vi "syncAIandAOat1MHz.vi"() -> ()   [LabVIEW 2015]
uses:
  <vilib>/DAQmx/write.llb/DAQmx Write (Digital 1D Wfm NChan NSamp).vi
  <vilib>/DAQmx/write.llb/DAQmx Write (Analog 1D Wfm NChan NSamp).vi
  <vilib>/DAQmx/read.llb/DAQmx Read (Analog 2D I16 NChan NSamp).vi
  <vilib>/Waveform/DWDTOps.llb/DWDT Analog to Digital.vi
  <vilib>/DAQmx/create/channels.llb/DAQmx Create Channel (AO-Voltage-Basic).vi
  <vilib>/DAQmx/create/channels.llb/DAQmx Create Channel (AI-Voltage-Basic).vi
  <vilib>/DAQmx/create/channels.llb/DAQmx Create Channel (DO-Digital Output).vi
  <vilib>/DAQmx/configure/timing.llb/DAQmx Timing (Sample Clock).vi
  <vilib>/Waveform/DWDTOps.llb/DWDT Uncompress Digital.vi
  <vilib>/DAQmx/miscellaneous.llb/DAQmx Fill In Error Info.vi
  <vilib>/DAQmx/configure/trigger.llb/DAQmx Start Trigger (Digital Edge).vi
  <resource>/objmgr/daqmx.rc
panel:
  in  "error in 3":errorcluster caption="error in"
  in  "index (page)":i32
  out "XY Graph":T1(graph)
  in  "V":dbl=2.0 format="%#_13g"
  in  "AOrate":dbl=400000.0 format="%#_13g"
  in  "stop":bool
  out "Intensity Graph":sgl[][](graph)
  in  "error in 2":errorcluster caption="error in"
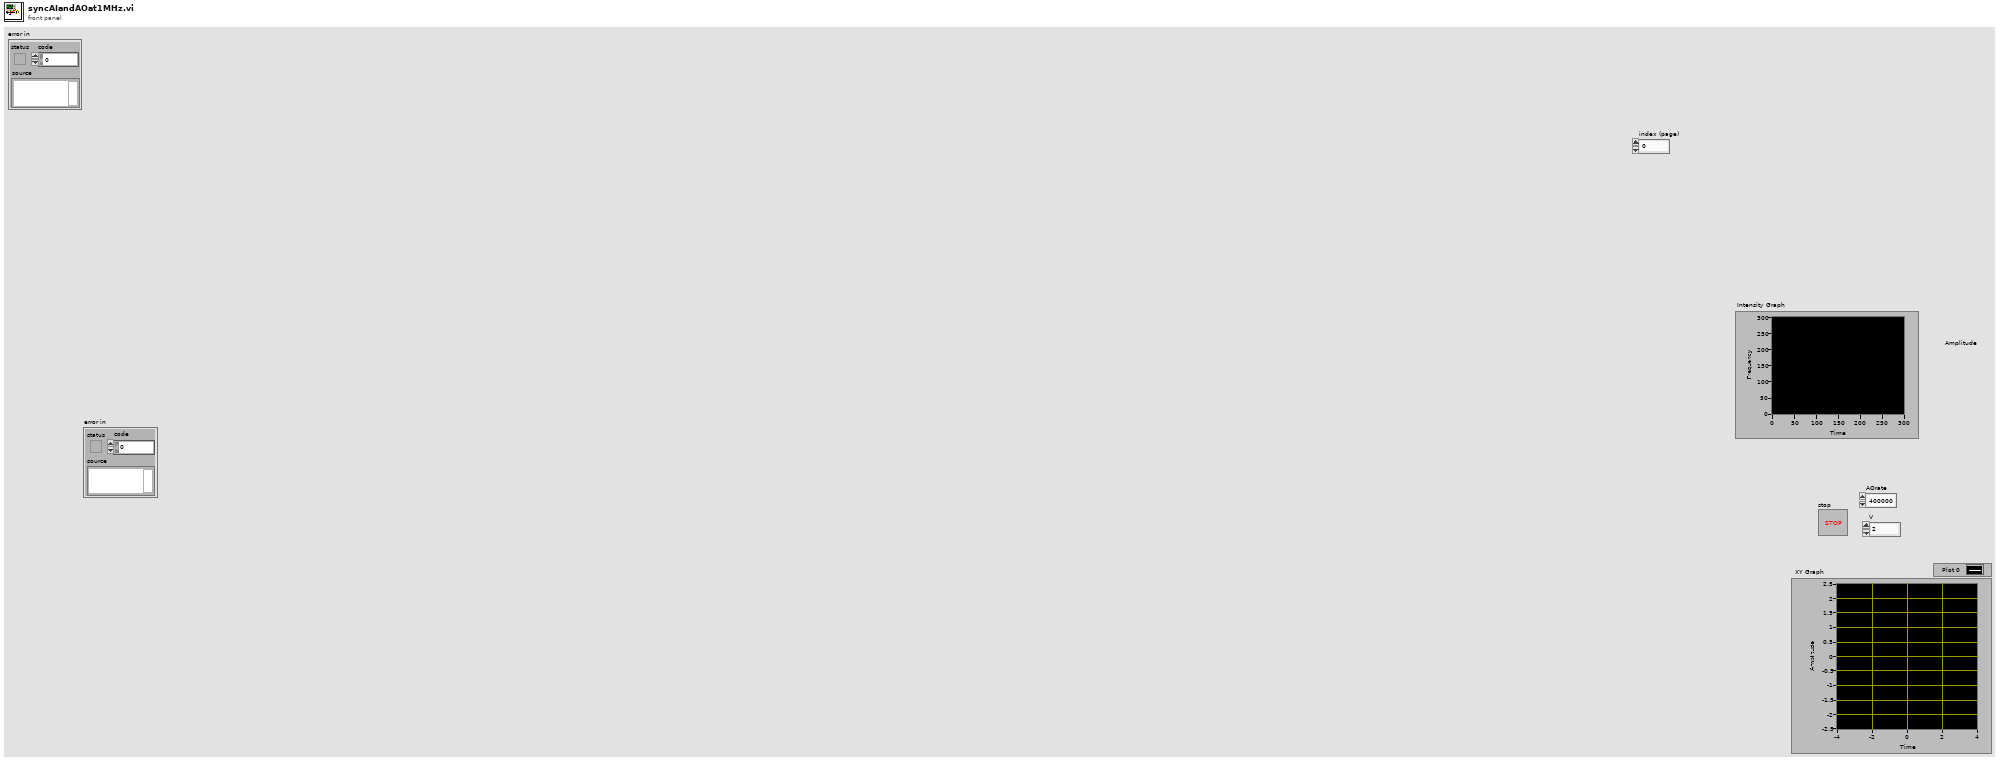
[diagram p1: front panel]
types:
  T1 = cluster{"X-WaveArray":dbl[], "Y-WaveArray":dbl[]}
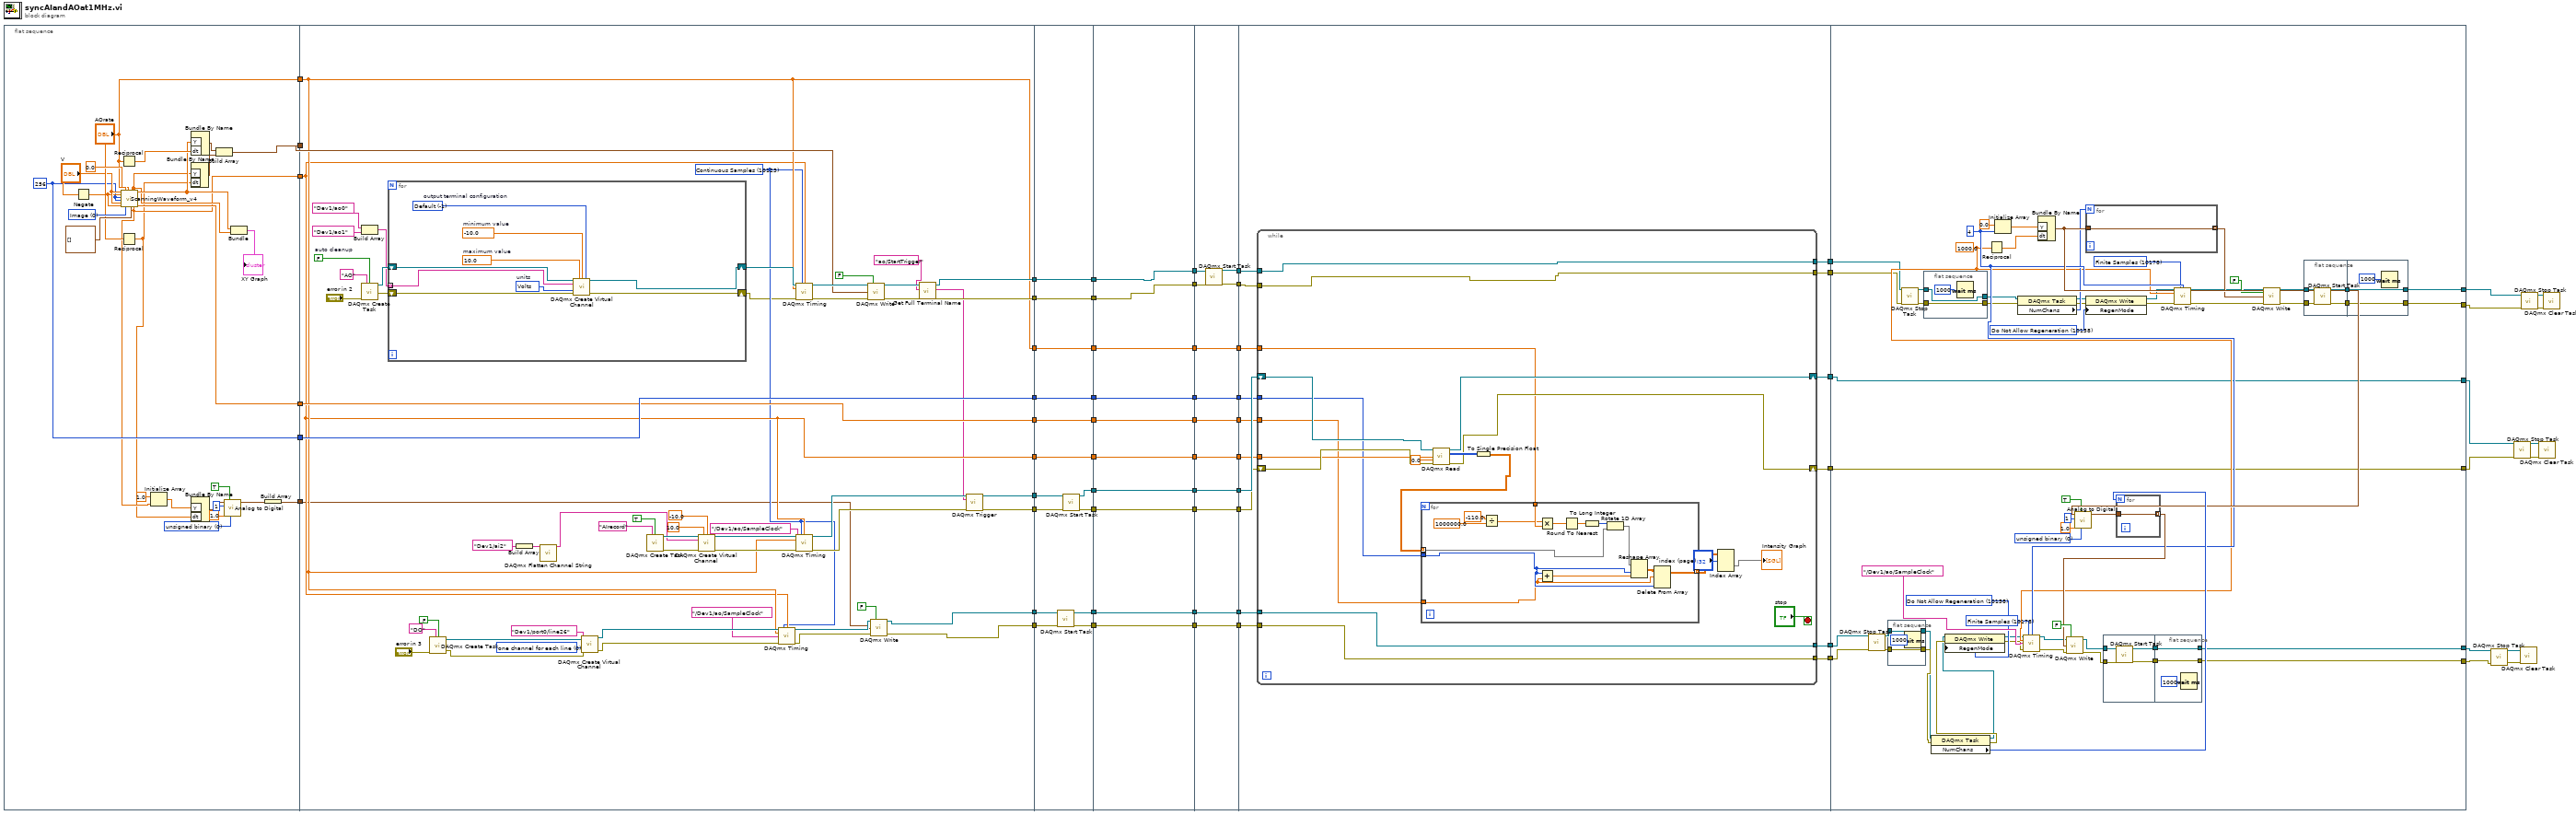
[diagram p0: block diagram]
diagram:
  n1 = flat-sequence {
    tunnel: [w79] -> w64
    tunnel: [w75] -> w63
    tunnel: ["AOrate"] -> w62
    tunnel: [w81] -> w38
    tunnel: [w80] -> w33
    tunnel: [w65] -> w17
    tunnel: w64 -> [w135]
    tunnel: w63 -> [w102]
    tunnel: w62 -> [w103]
    tunnel: [w117] -> w61
    tunnel: [w123] -> w58
    tunnel: [w121] -> w57
    tunnel: [w102] -> w43
    tunnel: [w103] -> w39
    tunnel: w38 -> [w125]
    tunnel: [w125] -> w34
    tunnel: w33 -> [w124]
    tunnel: [w124] -> w29
    tunnel: [w116] -> w28
    tunnel: [w94] -> w25
    tunnel: [w93] -> w24
    tunnel: w17 -> [w92]
    tunnel: w61 -> [w170]
    tunnel: [w170] -> w60
    tunnel: [w169] -> w59
    tunnel: w58 -> [w168]
    tunnel: w57 -> [w167]
    tunnel: [w166] -> w51
    tunnel: [w165] -> w49
    tunnel: [w164] -> w44
    tunnel: w43 -> [w164]
    tunnel: [w163] -> w40
    tunnel: w39 -> [w163]
    tunnel: [w162] -> w35
    tunnel: w34 -> [w162]
    tunnel: [w161] -> w30
    tunnel: w29 -> [w161]
    tunnel: w28 -> [w169]
    tunnel: w25 -> [w160]
    tunnel: w24 -> [w159]
    tunnel: [w158] -> w21
    tunnel: [w157] -> w18
    tunnel: w60 -> [w174]
    tunnel: w59 -> [w173]
    tunnel: [w174] -> w56
    tunnel: [w173] -> w54
    tunnel: [w180] -> w52
    tunnel: w51 -> [w180]
    tunnel: [w179] -> w50
    tunnel: w49 -> [w179]
    tunnel: [w178] -> w45
    tunnel: w44 -> [w178]
    tunnel: [w177] -> w41
    tunnel: w40 -> [w177]
    tunnel: [w176] -> w36
    tunnel: w35 -> [w176]
    tunnel: [w175] -> w31
    tunnel: w30 -> [w175]
    tunnel: [w172] -> w22
    tunnel: w21 -> [w172]
    tunnel: [w171] -> w19
    tunnel: w18 -> [w171]
    tunnel: w56 -> [w186]
    tunnel: [w184] -> w55
    tunnel: w54 -> [w185]
    tunnel: [w183] -> w53
    tunnel: w52 -> [w192]
    tunnel: w50 -> [w191]
    tunnel: [w192] -> w48
    tunnel: [w191] -> w47
    tunnel: [w190] -> w46
    tunnel: w45 -> [w190]
    tunnel: [w189] -> w42
    tunnel: w41 -> [w189]
    tunnel: [w188] -> w37
    tunnel: w36 -> [w188]
    tunnel: [w187] -> w32
    tunnel: w31 -> [w187]
    tunnel: [w182] -> w23
    tunnel: w22 -> [w182]
    tunnel: [w181] -> w20
    tunnel: w19 -> [w181]
    tunnel: w55 -> [w199]
    tunnel: w53 -> [w200]
    tunnel: w48 -> [w208]
    tunnel: w47 -> [w207]
    tunnel: w46 -> [w206]
    tunnel: w42 -> [w203]
    tunnel: w37 -> [w202]
    tunnel: w32 -> [w201]
    tunnel: w23 -> [w196]
    tunnel: w20 -> [w195]
    tunnel: [w205] -> w14
    tunnel: [w204] -> w13
    tunnel: [w198] -> w12
    tunnel: [w197] -> w11
    tunnel: [w194] -> w10
    tunnel: [w193] -> w9
    tunnel: w14 -> [w247]
    tunnel: w13 -> [w246]
    tunnel: w12 -> [w251]
    tunnel: w11 -> [w250]
    tunnel: w10 -> [w249]
    tunnel: w9 -> [w248]
    tunnel: [w247] -> w4
    tunnel: [w246] -> w3
    tunnel: [w245] -> w6
    tunnel: [w244] -> w5
    tunnel: [w243] -> w1
    tunnel: [w242] -> w2
    frame #0 {
      w67 = u16 0 items=["unsigned binary", "offset binary", "2's complement"] ("data format (offset binary)")
      w81 = 256
      w89 = u16 0 items=["Image", "Fill Rectangle", "Fill Circle", "Draw Freeform", "Fill Freeform", "Ellipse Boundary", "Line"] ("Drawing Mode")
      n2 = Negate(x="V") -> (-x=w82:dbl)
      n3 = Reciprocal(x="AOrate") -> (1/x=w87:dbl)
      n4 = Reciprocal(x="AOrate") -> (1/x=w72:dbl)
      n5 = call "ScanningWaveform_v4.vi"("Vy-min"=w82, "Vy-max"="V", "yPixels/tPixels"=w81, "xPixels/rPixels"=w81, "Vx-min"=w82, "Vx-max"="V", "Drawing Mode"=w89, "Angle"=0.0, "AOrate"="AOrate", "Points"=cluster{"X":dbl, "Y":dbl}[] []) -> ("numPixels"=w75:dbl, "Y-WaveArray"=w77:dbl[], "P"=w80:dbl, "X-WaveArray"=w78:dbl[])  [unwired: 6 in]
      n6 = Initialize Array(1.0 ("element"), w75) -> (w73:dbl[])
      n7 = Bundle By Name("Y"=w77, "dt"=w72) -> (w85:waveform(dbl))  [unwired: 1 in]
      n8 = Bundle By Name("Y"=w78, "dt"=w87) -> (w86:waveform(dbl))  [unwired: 1 in]
      n9 = Bundle By Name("Y"=w73, "dt"=w72) -> (w71:waveform(dbl))  [unwired: 1 in]
      n10 = Build Array(w86, w85) -> (w79:waveform(dbl)[])
      n11 = call-poly <vilib>:"Analog to Digital.vi"("data format (offset binary)"=w67, "compress digital (T)"=TRUE, "full-scale range (pk-pk)"=1.0, "resolution (16 bit)"=1, "analog waveform"=w71) -> ("digital waveform"=w66:digitalwaveform)  [unwired: 3 in, 3 out]
      n12 = Bundle("X-WaveArray"=w78, "Y-WaveArray"=w77) -> (→"XY Graph":T1)  [unwired: 1 in]
      n13 = Build Array(w66) -> (w65:digitalwaveform[])
    }
    frame #1 {
      w106 = 0 items=["one channel for each line", "one channel for all lines"] ("line grouping")
      w101 = 10123 items=["Finite Samples"=10178, "Continuous Samples"=10123, "Hardware Timed Single Point"=12522] ("sample mode")
      w145 = FALSE  # auto cleanup
      n14 = Build Array(tag "Dev1/ao0" ("physical channels"), tag "Dev1/ao1" ("physical channels")) -> (w136:tag[])
      n15 = call <vilib>:"DAQmx Create Task.vi"("new task name"="AO", "auto cleanup"=w145, "error in"="error in 2") -> ("task out"=w146:refnum<k21>, "error out"=w147:errorcluster)  [unwired: 11 in]
      n16 = for {
        shift-right: [w149] -> w142
        shift-left: w146 -> [w152]
        shift-right: [w148] -> w91
        shift-left: w147 -> [w151]
        tunnel: w136 -> [w150] mode=indexing
        w156 = -1 items=["Default"=-1, "RSE"=10083, "Differential"=10106, "Pseudodifferential"=12529]  # output terminal configuration
        w155 = 10348 items=["Volts"=10348, "From Custom Scale"=10065]  # units
        w154 = -10.0  # minimum value
        w153 = 10.0  # maximum value
        n17 = call-poly <vilib>:"DAQmx Create Virtual Channel.vi"("task in"=w152, "maximum value"=w153, "minimum value"=w154, "output terminal configuration"=w156, "physical channels"=w150, "units"=w155, "error in"=w151) -> ("task out"=w149:refnum<k21>, "error out"=w148:errorcluster)  [unwired: 7 in]
      }
      n18 = call <vilib>:"DAQmx Create Task.vi"("new task name"="DO", "auto cleanup"=FALSE, "error in"="error in 3") -> ("task out"=w110:refnum<k21>, "error out"=w105:errorcluster)  [unwired: 11 in]
      n19 = Build Array(tag "Dev1/ai2" ("physical channels")) -> (w114:tag[])
      n20 = call <vilib>:"DAQmx Flatten Channel String.vi"("names in"=w114) -> ("names out"=w112:string)  [unwired: 13 in, 1 out]
      n21 = call-poly <vilib>:"DAQmx Create Virtual Channel.vi"("task in"=w110, "lines"=tag "Dev1/port0/line26", "line grouping"=w106, "error in"=w105) -> ("task out"=w104:refnum<k21>, "error out"=w99:errorcluster)  [unwired: 10 in]
      n22 = call <vilib>:"DAQmx Create Task.vi"("new task name"="AIrecord", "auto cleanup"=TRUE) -> ("task out"=w128:refnum<k21>, "error out"=w129:errorcluster)  [unwired: 12 in]
      n23 = call-poly <vilib>:"DAQmx Create Virtual Channel.vi"("task in"=w128, "maximum value"=10.0, "minimum value"=-10.0, "physical channels"=w112, "error in"=w129) -> ("task out"=w134:refnum<k21>, "error out"=w133:errorcluster)  [unwired: 9 in]
      n24 = call-poly <vilib>:"DAQmx Timing.vi"("task/channels in"=w104, "sample mode"=w101, "samples per channel"=w102, "rate"=w103, "source"=tag "/Dev1/ao/SampleClock", "error in"=w99) -> ("task out"=w98:refnum<k21>, "error out"=w97:errorcluster)  [unwired: 8 in]
      n25 = call-poly <vilib>:"DAQmx Timing.vi"("task/channels in"=w134, "sample mode"=w101, "samples per channel"=w102, "rate"=w103, "source"=tag "/Dev1/ao/SampleClock", "error in"=w133) -> ("task out"=w126:refnum<k21>, "error out"=w122:errorcluster)  [unwired: 8 in]
      n26 = call-poly <vilib>:"DAQmx Timing.vi"("task/channels in"=w142, "sample mode"=w101, "samples per channel"=w102, "rate"=w103, "error in"=w91) -> ("task out"=w141:refnum<k21>, "error out"=w140:errorcluster)  [unwired: 2 in, 7 out]
      n27 = call-poly <vilib>:"DAQmx Write.vi"("task/channels in"=w141, "auto start"=FALSE, "data"=w135, "error in"=w140) -> ("task out"=w120:refnum<k21>, "error out"=w119:errorcluster)  [unwired: 9 in, 1 out]
      n28 = call-poly <vilib>:"DAQmx Write.vi"("task/channels in"=w98, "auto start"=FALSE, "data"=w92, "error in"=w97) -> ("task out"=w94:refnum<k21>, "error out"=w93:errorcluster)  [unwired: 9 in, 1 out]
      n29 = call "Get Full Terminal Name.vi"("error in"=w119, "Local Terminal Name"="ao/StartTrigger", "task/channels in"=w120) -> ("error out"=w116:errorcluster, "Terminal Name with Device Prefix"=w95:tag, "task out"=w117:refnum<k21>)  [unwired: 6 in]
      n30 = call-poly <vilib>:"DAQmx Trigger.vi"("task/channels in"=w126, "source"=w95, "error in"=w122) -> ("task out"=w123:refnum<k21>, "error out"=w121:errorcluster)  [unwired: 11 in]
    }
    frame #2 {
      n31 = call <vilib>:"DAQmx Start Task.vi"("task/channels in"=w160, "error in"=w159) -> ("task out"=w158:refnum<k21>, "error out"=w157:errorcluster)  [unwired: 12 in]
      n32 = call <vilib>:"DAQmx Start Task.vi"("task/channels in"=w168, "error in"=w167) -> ("task out"=w166:refnum<k21>, "error out"=w165:errorcluster)  [unwired: 12 in]
    }
    frame #3 {
    }
    frame #4 {
      n33 = call <vilib>:"DAQmx Start Task.vi"("task/channels in"=w186, "error in"=w185) -> ("task out"=w184:refnum<k21>, "error out"=w183:errorcluster)  [unwired: 12 in]
    }
    frame #5 {
      n34 = while {
        tunnel: w206 -> [w224]
        tunnel: w203 -> [w219]
        tunnel: w202 -> [w218]
        tunnel: w201 -> [w217]
        shift-right: [w222] -> w205
        shift-left: w208 -> [w226]
        shift-right: [w221] -> w204
        shift-left: w207 -> [w225]
        tunnel: w200 -> [w214]
        tunnel: w199 -> [w215]
        tunnel: [w215] -> w198
        tunnel: [w214] -> w197
        tunnel: w196 -> [w210]
        tunnel: w195 -> [w209]
        tunnel: [w210] -> w194
        tunnel: [w209] -> w193
        stop <- "stop" stop-if-true
        n35 = call-poly <vilib>:"DAQmx Read.vi"("task/channels in"=w226, "number of samples per channel"=w224, "timeout"=0.0, "error in"=w225) -> ("task out"=w222:refnum<k21>, "data"=w227:i16[][], "error out"=w221:errorcluster)  [unwired: 9 in]
        n36 = To Single Precision Float(number=w227) -> (single precision float=w220:sgl[][])
        n37 = for {
          tunnel: w220 -> [w241] mode=indexing
          tunnel: w219 -> [w240]
          tunnel: w218 -> [w239]
          tunnel: w217 -> [w238]
          tunnel: [w228] -> w213 mode=indexing
          n38 = Divide(x=-110.0, y=1000000.0) -> (x/y=w234:dbl)
          n39 = Multiply(x=w234, y=w240) -> (x*y=w230:dbl)
          n40 = Add(x=w239, y=w238) -> (x+y=w229:dbl)
          n41 = Round To Nearest(number=w230) -> (nearest integer value=w233:dbl)
          n42 = To Long Integer(number=w233) -> (32bit integer=w231:i32)
          n43 = Rotate 1D Array(1:w241, 2:w231) -> (0:w232:sgl[])
          n44 = Reshape Array(w232, w239, w229) -> (w237:sgl[][])
          n45 = Delete From Array(array=w237, length=w238, index (col)=w239) -> (array with subset deleted=w228:sgl[][])  [unwired: 1 in, 1 out]
        }
        n46 = Index Array(array=w213, index (dim 0)="index (page)") -> (element=→"Intensity Graph":sgl[][])  [unwired: 2 in]
      }
    }
    frame #6 {
      w277 = u16 0 items=["unsigned binary", "offset binary", "2's complement"] ("data format (offset binary)")
      w269 = 10178 items=["Finite Samples"=10178, "Continuous Samples"=10123, "Hardware Timed Single Point"=12522] ("sample mode")
      w272 = 10158 items=["Allow Regeneration"=10097, "Do Not Allow Regeneration"=10158] ("RegenMode")
      w280 = 1000.0 ("rate")
      w291 = 4 ("samples per channel")
      w255 = 10178 items=["Finite Samples"=10178, "Continuous Samples"=10123, "Hardware Timed Single Point"=12522] ("sample mode")
      w252 = 10158 items=["Allow Regeneration"=10097, "Do Not Allow Regeneration"=10158] ("RegenMode")
      n47 = call <vilib>:"DAQmx Stop Task.vi"("task/channels in"=w249, "error in"=w248) -> ("task out"=w264:refnum<k21>, "error out"=w263:errorcluster)  [unwired: 12 in]
      n48 = flat-sequence {
        tunnel: w264 -> [w306]
        tunnel: [w306] -> w286
        tunnel: w263 -> [w305]
        tunnel: [w305] -> w288
        frame #0 {
          n49 = Wait (ms)(milliseconds to wait=u32 1000) -> ()  [unwired: 1 out]
        }
      }
      n50 = call <vilib>:"DAQmx Stop Task.vi"("task/channels in"=w251, "error in"=w250) -> ("task out"=w260:refnum<k21>, "error out"=w261:errorcluster)  [unwired: 12 in]
      n51 = flat-sequence {
        tunnel: w260 -> [w316]
        tunnel: [w316] -> w262
        tunnel: w261 -> [w315]
        tunnel: [w315] -> w282
        frame #0 {
          n52 = Wait (ms)(milliseconds to wait=u32 1000) -> ()  [unwired: 1 out]
        }
      }
      n53 = property class="DAQmx Task"(reference=w286, error in=w288) -> (reference out=w287:refnum<k21>, error out=w289:errorcluster, "NumChans"=w294:u32)
      n54 = property class="DAQmx Write"(reference=w287, error in=w289, "RegenMode"=w272) -> (reference out=w271:refnum<k21>, error out=w270:errorcluster)
      n55 = Reciprocal(x=w280) -> (1/x=w290:dbl)
      n56 = Initialize Array(0.0 ("element"), w291) -> (w278:dbl[])
      n57 = property class="DAQmx Task"(reference=w262, error in=w282) -> (reference out=w281:refnum<k21>, error out=w283:errorcluster, "NumChans"=w285:u32)
      n58 = call-poly <vilib>:"DAQmx Timing.vi"("task/channels in"=w271, "sample mode"=w269, "samples per channel"=w291, "rate"=w280, "source"=tag "/Dev1/ao/SampleClock", "error in"=w270) -> ("task out"=w268:refnum<k21>, "error out"=w267:errorcluster)  [unwired: 8 in]
      n59 = Bundle By Name("Y"=w278, "dt"=w290) -> (w292:waveform(dbl))  [unwired: 1 in]
      n60 = call-poly <vilib>:"Analog to Digital.vi"("data format (offset binary)"=w277, "compress digital (T)"=TRUE, "full-scale range (pk-pk)"=1.0, "resolution (16 bit)"=1, "analog waveform"=w292) -> ("digital waveform"=w293:digitalwaveform)  [unwired: 3 in, 3 out]
      n61 = for {
        N: w285 -> [_]
        tunnel: w292 -> [w303]
        tunnel: [w303] -> w284 mode=indexing
      }
      n62 = property class="DAQmx Write"(reference=w281, error in=w283, "RegenMode"=w252) -> (reference out=w253:refnum<k21>, error out=w254:errorcluster)
      n63 = flat-sequence {
        tunnel: [w308] -> w299
        tunnel: [w307] -> w298
        tunnel: w266 -> [w310]
        tunnel: w265 -> [w309]
        tunnel: [w312] -> w243
        tunnel: [w313] -> w242
        tunnel: w299 -> [w313]
        tunnel: w298 -> [w312]
        frame #0 {
          n64 = call <vilib>:"DAQmx Start Task.vi"("task/channels in"=w310, "error in"=w309) -> ("task out"=w308:refnum<k21>, "error out"=w307:errorcluster)  [unwired: 12 in]
        }
        frame #1 {
          n65 = Wait (ms)(milliseconds to wait=u32 1000) -> ()  [unwired: 1 out]
        }
      }
      n66 = for {
        N: w294 -> [_]
        tunnel: w293 -> [w302]
        tunnel: [w302] -> w295 mode=indexing
      }
      n67 = call-poly <vilib>:"DAQmx Write.vi"("task/channels in"=w268, "auto start"=FALSE, "data"=w295, "error in"=w267) -> ("task out"=w266:refnum<k21>, "error out"=w265:errorcluster)  [unwired: 9 in, 1 out]
      n68 = call-poly <vilib>:"DAQmx Timing.vi"("task/channels in"=w253, "sample mode"=w255, "samples per channel"=w291, "rate"=w280, "error in"=w254) -> ("task out"=w256:refnum<k21>, "error out"=w257:errorcluster)  [unwired: 9 in]
      n69 = call-poly <vilib>:"DAQmx Write.vi"("task/channels in"=w256, "auto start"=FALSE, "data"=w284, "error in"=w257) -> ("task out"=w258:refnum<k21>, "error out"=w259:errorcluster)  [unwired: 9 in, 1 out]
      n70 = flat-sequence {
        tunnel: [w318] -> w301
        tunnel: [w317] -> w300
        tunnel: w258 -> [w320]
        tunnel: w259 -> [w319]
        tunnel: [w322] -> w244
        tunnel: [w323] -> w245
        tunnel: w301 -> [w323]
        tunnel: w300 -> [w322]
        frame #0 {
          n71 = call <vilib>:"DAQmx Start Task.vi"("task/channels in"=w320, "error in"=w319) -> ("task out"=w318:refnum<k21>, "error out"=w317:errorcluster)  [unwired: 12 in]
        }
        frame #1 {
          n72 = Wait (ms)(milliseconds to wait=u32 1000) -> ()  [unwired: 1 out]
        }
      }
    }
  }
  n73 = call <vilib>:"DAQmx Stop Task.vi"("task/channels in"=w2, "error in"=w1) -> ("task out"=w15:refnum<k21>, "error out"=w16:errorcluster)  [unwired: 12 in]
  n74 = call <vilib>:"DAQmx Stop Task.vi"("task/channels in"=w4, "error in"=w3) -> ("task out"=w8:refnum<k21>, "error out"=w7:errorcluster)  [unwired: 12 in]
  n75 = call <vilib>:"DAQmx Clear Task.vi"("task in"=w15, "error in"=w16) -> ()  [unwired: 13 in, 1 out]
  n76 = call <vilib>:"DAQmx Stop Task.vi"("task/channels in"=w6, "error in"=w5) -> ("task out"=w27:refnum<k21>, "error out"=w26:errorcluster)  [unwired: 12 in]
  n77 = call <vilib>:"DAQmx Clear Task.vi"("task in"=w8, "error in"=w7) -> ()  [unwired: 13 in, 1 out]
  n78 = call <vilib>:"DAQmx Clear Task.vi"("task in"=w27, "error in"=w26) -> ()  [unwired: 13 in, 1 out]
